vi "MAX_CameraSend Images To PC Loop.vi"(8 "error in (no error)":errorcluster) -> ()   [LabVIEW 2016]
doc: "This VI is used to send images to the dashboard using the second enet port on the 8 slot controller. This is provided for compatibility, but is higher overhead than using the Camera MJPG approach.\n\nThis software is licensed. Open the labview\\readme\\WPI Robotics Library Open Source License.txt file for more information."
uses:
  <vilib>/Rock Robotics/WPI/Utilities/Refnum Registry Operation.ctl
  <vilib>/Rock Robotics/Network Tables/NT Write String Array.vi
  <vilib>/Rock Robotics/Network Tables/NT Write String.vi
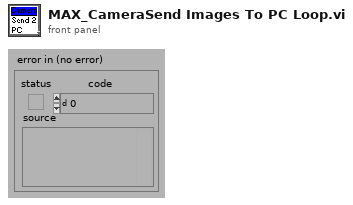
[diagram p1: front panel]
types:
  T1 = enum16{"Standard", "Buffered", "CRLF", "Immediate"}
  T2 = typedef "Refnum Registry Operation.ctl" = enum16{"set", "get", "delete", "get all names", "read name"}
  T3 = cluster{"token string":string, "token string 2":string}[]
  T4 = typedef "WPI_CameraDevRef.ctl" = cluster{"Camera Address":string, "CameraStatus":errorcluster}
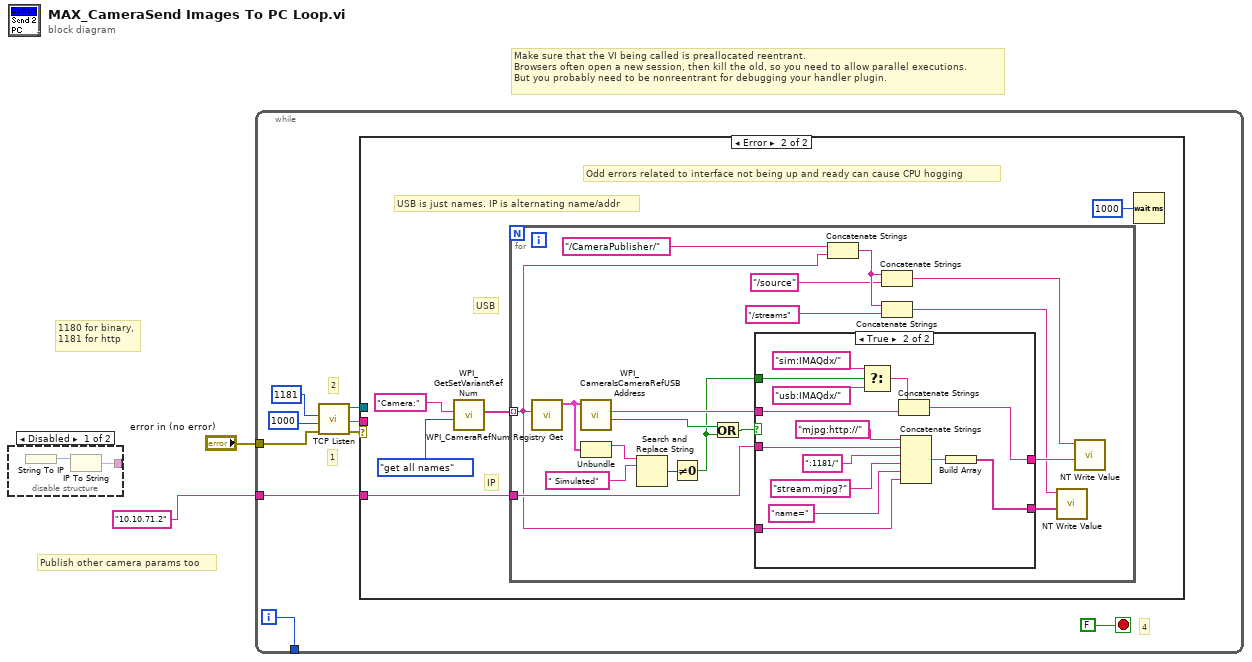
[diagram p0: block diagram]
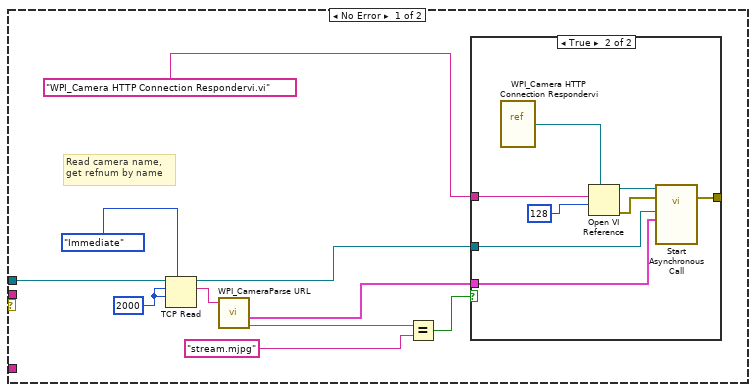
[diagram p3: hidden frame]
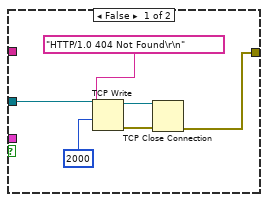
[diagram p4: hidden frame]
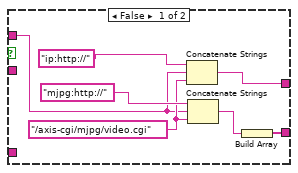
[diagram p5: hidden frame]
diagram:
  # "Make sure that the VI being called is preallocated reentrant.\nBrowsers often open a new session, then kill the old, so you need to allow parallel executions.\nBut you probably need to be nonreentrant for debugging your handler plugin."
  # "Publish other camera params too"
  # "1180 for binary,\n1181 for http"
  n1 = disable-structure shown="Disabled" {
    disable-tunnel: [w4 _] -> _
    frame Disabled {
      n2 = String To IP() -> (0:w3:u32)  [unwired: 1 in]
      n3 = IP To String(2:w3) -> (0:w4:string)  [unwired: 1 in]
    }
    frame Enabled {
    }
  }
  n4 = while {
    tunnel: "error in (no error)" -> [w12]
    tunnel: [w7] -> _
    tunnel: "10.10.71.2" ("name") -> [w5]
    i -> [w7]
    stop <- FALSE ("status") stop-if-true
    # "4"
    # "1"
    # "2"
    n5 = call <vilib>:"TCP Listen.vi"("error in (no error)"=w12, "timeout ms (wait forever: -1)"=u16 1000 ("port"), "port"=u16 1181) -> ("error out"=w9:errorcluster, "remote address"=w13:string, "connection ID"=w11:refnum<k5>)  [unwired: 1 in, 5 out]
    n6 = case shown="Error" w9 {
      tunnel: w13 -> [_ _]
      tunnel: w11 -> [w20 _]
      tunnel: w5 -> [_ w38]
      frame No Error {
        w21 = 2000
        # "Read camera name,\nget refnum by name"
        n7 = TCP Read(connection ID=w20, bytes to read=w21, 7:T1."Immediate" ("mode (standard)"), 9:w21) -> (connection ID out=w19:refnum<k5>, data out=w14:string)  [unwired: 1 in, 1 out]
        n8 = call <vilib>:"WPI_CameraParse URL.vi"("URL"=w14) -> ("cgi string"=w16:string, "parameters"=w15:T3)  [unwired: 7 in, 2 out]
        n9 = Equal?(x=w16, y="stream.mjpg") -> (x = y?=w18:bool)
        n10 = case shown="True" w18 {
          tunnel: "WPI_Camera HTTP Connection Respondervi.vi" -> [_ w37]
          tunnel: w19 -> [w29 w33]
          tunnel: [w24 w31] -> _
          tunnel: w15 -> [_ w30]
          frame False {
            n11 = TCP Write(connection ID=w29, data in="HTTP/1.0 404 Not Found\r\n" ("regular expression"), 9:2000) -> (connection ID out=w28:refnum<k5>, error out=w25:errorcluster)  [unwired: 1 in, 1 out]
            n12 = TCP Close Connection(connection ID=w28, error in (no error)=w25) -> (error out=w24:errorcluster)  [unwired: 2 out]
          }
          frame True {
            n13 = vi-ref <vilib>:"WPI_Camera HTTP Connection Respondervi.vi"() -> (w35:refnum<vi>)
            n14 = Open VI Reference(type specifier VI Refnum (for type only)=w35, vi path=w37, options=128) -> (vi reference=w34:refnum<vi>, error out=w32:errorcluster)  [unwired: 3 in]
            n15 = call-by-ref "Start Asynchronous Call"(reference=w34, error in=w32, "parameters"=w30, "connection ID"=w33) -> (error out=w31:errorcluster)  [unwired: 10 in, 1 out]
          }
        }
      }
      frame Error {
        # "USB is just names. IP is alternating name/addr"
        # "IP"
        # "USB"
        # "Odd errors related to interface not being up and ready can cause CPU hogging"
        n16 = call <vilib>:"WPI_GetSetVariantRefNum.vi"("Operation"=Refnum_Registry_Operation."get all names" ("menu"), "refnum name"="Camera:") -> ("names"=w39:string[])  [unwired: 7 in, 2 out]
        n17 = for {
          tunnel: w39 -> [w57] mode=indexing
          tunnel: w38 -> [w60]
          n18 = call <vilib>:"WPI_CameraRefNum Registry Get.vi"("refnum name"=w57) -> ("CameraDevRef"=w48:T4)  [unwired: 9 in, 1 out]
          n19 = call <vilib>:"WPI_CameraIsCameraRefUSBAddress.vi"("CameraDevRef"=w48) -> ("USB?"=w45:bool, "Camera Address Out"=w50:string)  [unwired: 7 in, 2 out]
          n20 = Unbundle(w48) -> ("Camera Address"=w47:string)  [unwired: 1 out]
          n21 = Search and Replace String(input string=w47, search string=" Simulated") -> (number of replacements=w46:i32)  [unwired: 6 in, 3 out]
          n22 = Not Equal To 0?(x=w46) -> (x != 0?=w43:bool)
          n23 = Or(x=w45, y=w43) -> (x .or. y?=w44:bool)
          n24 = case shown="True" w44 {
            tunnel: w50 -> [w63 w73]
            tunnel: w60 -> [_ w80]
            tunnel: w57 -> [_ w76]
            tunnel: [w61 w72] -> w59
            tunnel: [w65 w74] -> w51
            tunnel: w43 -> [_ w71]
            frame False {
              w64 = "/axis-cgi/mjpg/video.cgi"
              n25 = Concatenate Strings("ip:http://", w63, w64) -> (w61:string)
              n26 = Concatenate Strings("mjpg:http://", w63, w64) -> (w66:string)
              n27 = Build Array(w66) -> (w65:string[])
            }
            frame True {
              n28 = Select(t="sim:IMAQdx/", s=w71, f="usb:IMAQdx/") -> (s? t:f=w68:string)
              n29 = Concatenate Strings(w68, w73) -> (w72:string)
              n30 = Concatenate Strings("mjpg:http://", w80, ":1181/", "stream.mjpg?", "name=", w76) -> (w75:string)
              n31 = Build Array(w75) -> (w74:string[])
            }
          }
          n32 = Concatenate Strings("/CameraPublisher/", w57) -> (w55:string)
          n33 = Concatenate Strings(w55, "/source") -> (w52:string)
          n34 = Concatenate Strings(w55, "/streams") -> (w53:string)
          n35 = call-poly <vilib>:"NT Write Value.vi"("String Array"=w51, "Name"=w53) -> ()  [unwired: 9 in, 1 out]
          n36 = call-poly <vilib>:"NT Write Value.vi"("String"=w59, "Name"=w52) -> ()  [unwired: 9 in, 1 out]
        }
        n37 = Wait (ms)(milliseconds to wait=u32 1000) -> ()  [unwired: 1 out]
      }
    }
  }
